vi "move to 2nd screen.vi"   [LabVIEW 2011]
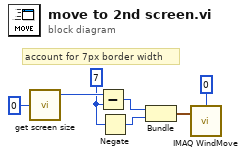
[diagram p0: block diagram]
diagram:
  w3 = i16 7 ("y")
  # "account for 7px border width"
  n1 = call "get screen size.vi"("screen"=0) -> ("width"=w6:i16)  [unwired: 2 in, 2 out]
  n2 = Subtract(x=w6, y=w3) -> (x-y=w5:i16)
  n3 = Negate(x=w3) -> (-x=w2:i16)
  n4 = Bundle(w5, w2) -> (w4:cluster{i16, i16})  [unwired: 1 in]
  n5 = call "IMAQ WindMove"("Window Number (0...15)"=0, "Coordinates (screen)"=w4) -> ()  [unwired: 3 in, 2 out]
